vi "Emballge_BDD_Lecture_balises_PPXml.vi"(8 "entrée d'erreur (pas d'erreur)":errorcluster, 11 "appended path":path) -> (0 "sortie d'erreur":errorcluster, 1 "Nb_valve_par_carton":string, 3 "affiche_code_barre_client":string, 4 "melange_des_lots_possible":string, 5 "Code_Barre_Fixe":string, 7 "Indice":string)   [LabVIEW 2020]
panel:
  out "x-y":u32
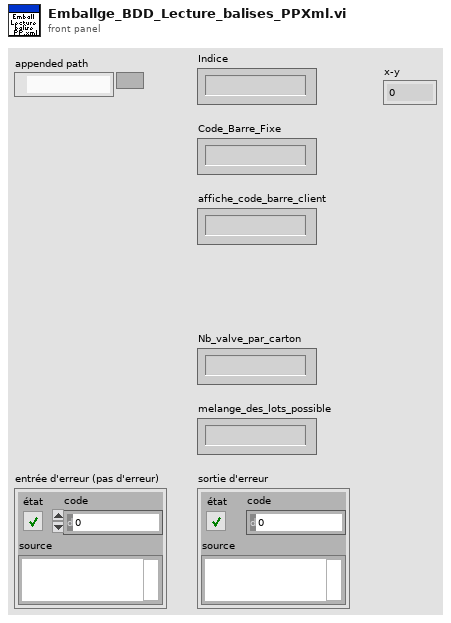
[diagram p1: front panel]
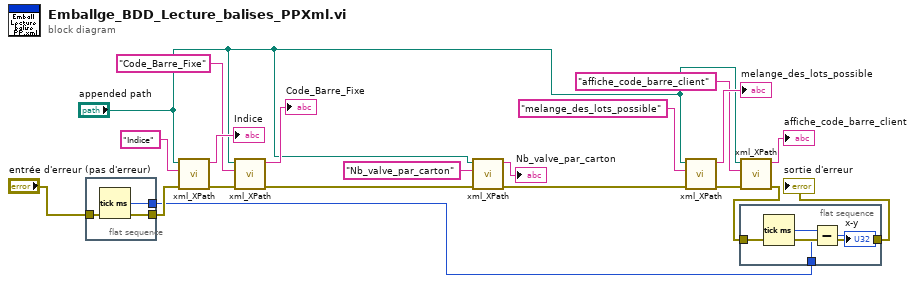
[diagram p0: block diagram]
diagram:
  n1 = flat-sequence {
    tunnel: [w22] -> w4
    tunnel: "entrée d'erreur (pas d'erreur)" -> [w22]
    tunnel: [w21] -> w1
    frame #0 {
      n2 = Tick Count (ms)() -> (millisecond timer value=w21:u32)
    }
  }
  n3 = call "xml_XPath.vi"("error in (no error)"=w4, "XPath expression"="Indice", "path to XML document"="appended path") -> ("sortie d'erreur"=w14:errorcluster, "valeur"=→"Indice":string)  [unwired: 3 in, 4 out]
  n4 = call "xml_XPath.vi"("error in (no error)"=w14, "XPath expression"="Code_Barre_Fixe", "path to XML document"="appended path") -> ("sortie d'erreur"=w8:errorcluster, "valeur"=→"Code_Barre_Fixe":string)  [unwired: 3 in, 4 out]
  n5 = call "xml_XPath.vi"("error in (no error)"=w8, "XPath expression"="Nb_valve_par_carton", "path to XML document"="appended path") -> ("sortie d'erreur"=w15:errorcluster, "valeur"=→"Nb_valve_par_carton":string)  [unwired: 3 in, 4 out]
  n6 = call "xml_XPath.vi"("error in (no error)"=w15, "XPath expression"="melange_des_lots_possible", "path to XML document"="appended path") -> ("sortie d'erreur"=w16:errorcluster, "valeur"=→"melange_des_lots_possible":string)  [unwired: 3 in, 4 out]
  n7 = flat-sequence {
    tunnel: [w26] -> w2
    tunnel: w3 -> [w26]
    tunnel: w1 -> [w23]
    frame #0 {
      n8 = Tick Count (ms)() -> (millisecond timer value=w25:u32)
      n9 = Subtract(x=w25, y=w23) -> (x-y=→"x-y":u32)
    }
  }
  n10 = call "xml_XPath.vi"("error in (no error)"=w16, "XPath expression"="affiche_code_barre_client", "path to XML document"="appended path") -> ("sortie d'erreur"=w3:errorcluster, "valeur"=→"affiche_code_barre_client":string)  [unwired: 3 in, 4 out]
  "sortie d'erreur" <- w2
